vi "Advanced Binding Test.vi"() -> (0 "error out":errorcluster)   [LabVIEW 2014, in "SQLite3LV Tests.lvlib"]
uses:
  SQLite3LV Tests.lvlib
  SQLite3LV/Cursor Class/property binding/bind text.vi
  SQLite3LV/Cursor Class/property binding/column I32.vi
  SQLite3LV/SQLite3 Class/sqlite3.lvclass
  SQLite3LV/Cursor Class/cursor.lvclass
panel:
  out "table count":i32
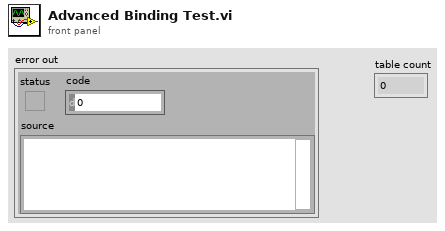
[diagram p1: front panel]
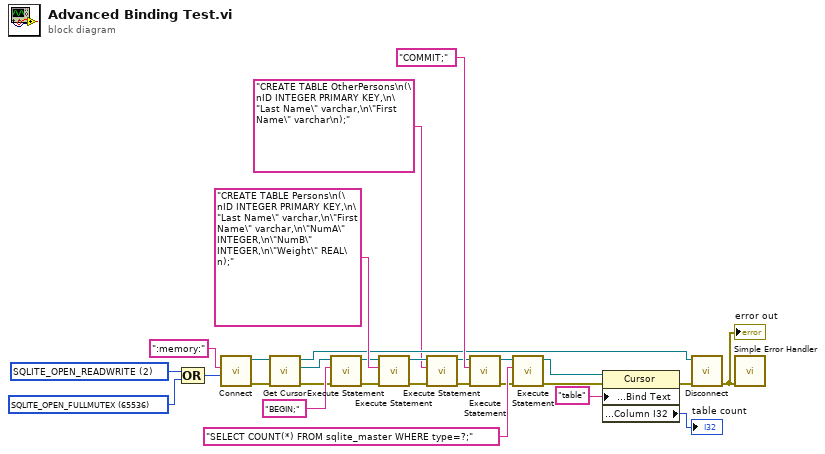
[diagram p0: block diagram]
diagram:
  w27 = u32 65536 items=["SQLITE_OPEN_READONLY"=1, "SQLITE_OPEN_READWRITE"=2, "SQLITE_OPEN_CREATE"=4, "SQLITE_OPEN_DELETEONCLOSE"=8, "SQLITE_OPEN_EXCLUSIVE"=16, "SQLITE_OPEN_AUTOPROXY"=32, "SQLITE_OPEN_URI"=64, "SQLITE_OPEN_MEMORY"=128, "SQLITE_OPEN_MAIN_DB"=256, "SQLITE_OPEN_TEMP_DB"=512, "SQLITE_OPEN_TRANSIENT_DB"=1024, "SQLITE_OPEN_MAIN_JOURNAL"=2048, "SQLITE_OPEN_TEMP_JOURNAL"=4096, "SQLITE_OPEN_SUBJOURNAL"=8192, "SQLITE_OPEN_MASTER_JOURNAL"=16384, "SQLITE_OPEN_NOMUTEX"=32768, "SQLITE_OPEN_FULLMUTEX"=65536, "SQLITE_OPEN_SHAREDCACHE"=131072, "SQLITE_OPEN_PRIVATECACHE"=262144, "SQLITE_OPEN_WAL"=524288] ("SQLITE3 Open Flag")
  w28 = u32 2 items=["SQLITE_OPEN_READONLY"=1, "SQLITE_OPEN_READWRITE"=2, "SQLITE_OPEN_CREATE"=4, "SQLITE_OPEN_DELETEONCLOSE"=8, "SQLITE_OPEN_EXCLUSIVE"=16, "SQLITE_OPEN_AUTOPROXY"=32, "SQLITE_OPEN_URI"=64, "SQLITE_OPEN_MEMORY"=128, "SQLITE_OPEN_MAIN_DB"=256, "SQLITE_OPEN_TEMP_DB"=512, "SQLITE_OPEN_TRANSIENT_DB"=1024, "SQLITE_OPEN_MAIN_JOURNAL"=2048, "SQLITE_OPEN_TEMP_JOURNAL"=4096, "SQLITE_OPEN_SUBJOURNAL"=8192, "SQLITE_OPEN_MASTER_JOURNAL"=16384, "SQLITE_OPEN_NOMUTEX"=32768, "SQLITE_OPEN_FULLMUTEX"=65536, "SQLITE_OPEN_SHAREDCACHE"=131072, "SQLITE_OPEN_PRIVATECACHE"=262144, "SQLITE_OPEN_WAL"=524288] ("SQLITE3 Open Flag")
  n1 = Compound Arithmetic op=OR(w28, w27) -> (w25:u32)
  n2 = call "Connect.vi"("SQLITE3 open flags"=w25, "path"=":memory:" ("path_utf8")) -> ("error out"=w23:errorcluster, "SQLite3LV Connection out"=w24:refnum<class "sqlite3.lvclass">)  [unwired: 8 in]
  n3 = call "Get Cursor.vi"("error in (no error)"=w23, "SQLite3LV Connection in"=w24) -> ("error out"=w14:errorcluster, "SQLite3LV Cursor"=w15:refnum<class "cursor.lvclass">, "SQLite3LV Connection out"=w17:refnum<class "sqlite3.lvclass">)  [unwired: 7 in]
  n4 = call "Execute Statement.vi"("error in (no error)"=w14, "SQL statement"="BEGIN;", "SQLite3LV Cursor in"=w15) -> ("error out"=w12:errorcluster, "SQLite3LV Cursor out"=w13:refnum<class "cursor.lvclass">)  [unwired: 7 in]
  n5 = call "Execute Statement.vi"("error in (no error)"=w12, "SQL statement"="CREATE TABLE Persons\n(\nID INTEGER PRIMARY KEY,\n\"Last Name\" varchar,\n\"First Name\" varchar,\n\"NumA\" INTEGER,\n\"NumB\" INTEGER,\n\"Weight\" REAL\n);" ("statement"), "SQLite3LV Cursor in"=w13) -> ("error out"=w10:errorcluster, "SQLite3LV Cursor out"=w11:refnum<class "cursor.lvclass">)  [unwired: 7 in]
  n6 = call "Execute Statement.vi"("error in (no error)"=w10, "SQL statement"="CREATE TABLE OtherPersons\n(\nID INTEGER PRIMARY KEY,\n\"Last Name\" varchar,\n\"First Name\" varchar\n);" ("statement"), "SQLite3LV Cursor in"=w11) -> ("error out"=w7:errorcluster, "SQLite3LV Cursor out"=w8:refnum<class "cursor.lvclass">)  [unwired: 7 in]
  n7 = call "Execute Statement.vi"("error in (no error)"=w7, "SQL statement"="COMMIT;", "SQLite3LV Cursor in"=w8) -> ("error out"=w6:errorcluster, "SQLite3LV Cursor out"=w5:refnum<class "cursor.lvclass">)  [unwired: 7 in]
  n8 = call "Execute Statement.vi"("error in (no error)"=w6, "SQL statement"="SELECT COUNT(*) FROM sqlite_master WHERE type=?;" ("statement"), "SQLite3LV Cursor in"=w5) -> ("error out"=w4:errorcluster, "SQLite3LV Cursor out"=w18:refnum<class "cursor.lvclass">)  [unwired: 7 in]
  n9 = property class="Cursor"(reference=w18, error in=w4, "property binding:Bind Text"="table" ("Bind Text")) -> (error out=w1:errorcluster, "property binding:Column I32"=→"table count":i32)  [unwired: 1 out]
  n10 = call "Disconnect.vi"("error in (no error)"=w1, "SQLite3LV Connection in"=w17) -> ("error out"=w20:errorcluster)  [unwired: 9 in]
  "error out" <- w20
  n11 = call <vilib>:"Simple Error Handler.vi"("error in (no error)"=w20) -> ()  [unwired: 4 in, 5 out]
